vi "Accumulate XY data.vi"(6 "max size":i32=4096, 7 "reset":bool, 11 "plots":cluster{"Y":dbl[], dbl[]}[](array[cluster])) -> (3 "plots out":cluster{dbl[], dbl[]}[](array[cluster]))   [LabVIEW 2013]
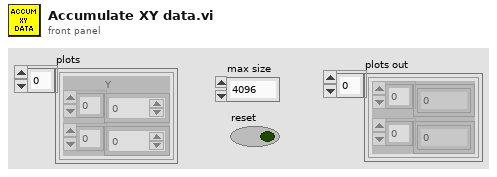
[diagram p1: front panel]
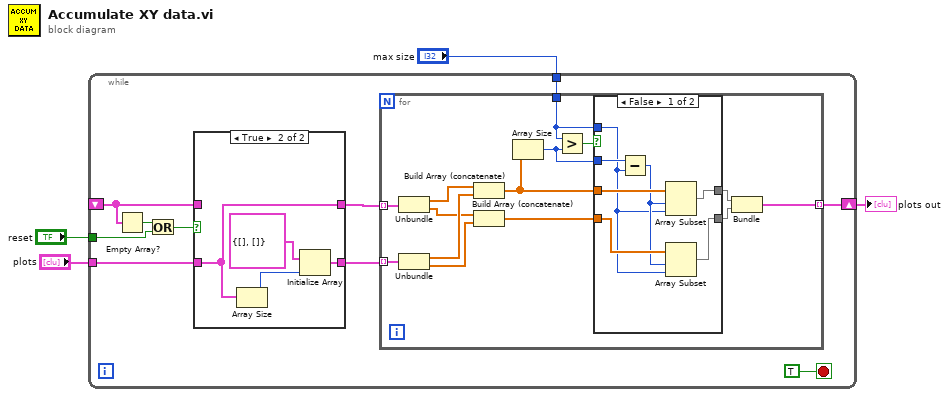
[diagram p0: block diagram]
diagram:
  n1 = while {
    tunnel: "plots" -> [w12]
    shift-right: [w14] -> w1
    shift-left: _ -> [w13]
    tunnel: "reset" -> [w7]
    tunnel: "max size" -> [w5]
    stop <- TRUE stop-if-true
    n2 = Empty Array?(array=w13) -> (empty?=w9:bool)
    n3 = Or(x=w9, y=w7) -> (x .or. y?=w8:bool)
    n4 = case shown="True" w8 {
      tunnel: w13 -> [w16 _]
      tunnel: w12 -> [w15 w20]
      tunnel: [w16 w20] -> w11
      tunnel: [w15 w17] -> w10
      frame False {
      }
      frame True {
        n5 = Array Size(array=w20) -> (size(s)=w19:i32)
        n6 = Initialize Array(cluster{dbl[], dbl[]} {[], []} ("output cluster"), w19) -> (w17:cluster{dbl[], dbl[]}[])
      }
    }
    n7 = for {
      tunnel: w11 -> [w34] mode=indexing
      tunnel: w10 -> [w33] mode=indexing
      tunnel: [w28] -> w14 mode=indexing
      tunnel: w5 -> [w22]
      n8 = Unbundle(w34) -> ("Y"=w32:dbl[], w30:dbl[])
      n9 = Unbundle(w33) -> ("Y"=w31:dbl[], w29:dbl[])
      n10 = Build Array (concatenate)(w32, w31) -> (w26:dbl[])
      n11 = Build Array (concatenate)(w30, w29) -> (w25:dbl[])
      n12 = Array Size(array=w26) -> (size(s)=w21:i32)
      n13 = Greater?(x=w22, y=w21) -> (0:w27:bool)
      n14 = case shown="False" w27 {
        tunnel: w26 -> [w40 w43]
        tunnel: [w36 w43] -> w23
        tunnel: w25 -> [w39 w42]
        tunnel: [w35 w42] -> w24
        tunnel: w22 -> [w37 _]
        tunnel: w21 -> [w41 _]
        frame False {
          n15 = Subtract(x=w41, y=w37) -> (x-y=w38:i32)
          n16 = Array Subset(array=w40, index=w38, length=w37) -> (w36:dbl[])
          n17 = Array Subset(array=w39, index=w38, length=w37) -> (w35:dbl[])
        }
        frame True {
        }
      }
      n18 = Bundle(w23, w24) -> (w28:cluster{dbl[], dbl[]})  [unwired: 1 in]
    }
  }
  "plots out" <- w1
